vi "Find All New VIs.vi"(8 "error in":errorcluster, 10 "VIs  to exclude":variant) -> (0 "error out":errorcluster, 3 "VI refs":refnum<vi>[](array[refnum]))   [LabVIEW 2012, in "NI_SE_Config Front Panel Layout.lvlib"]
doc: "Find all VIs in memory that can be added to the layout configuration."
uses:
  NI_SE_Config Front Panel Layout.lvlib
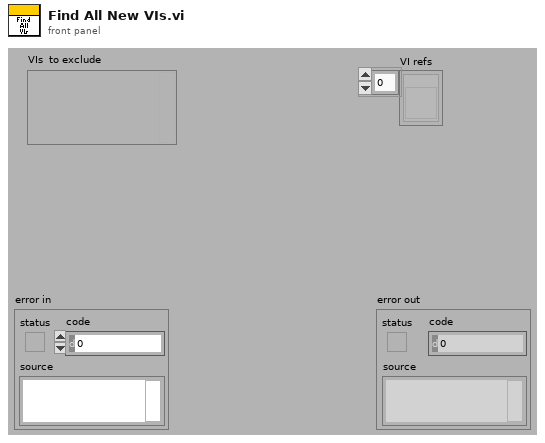
[diagram p1: front panel]
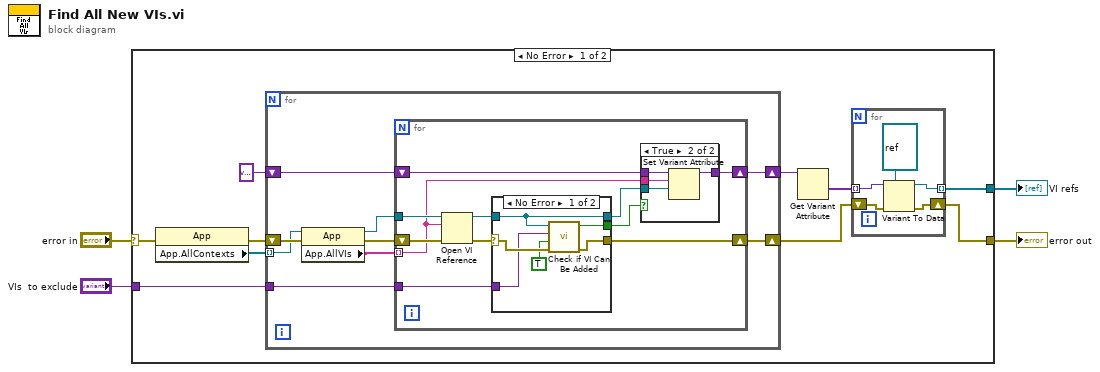
[diagram p0: block diagram]
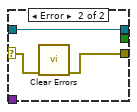
[diagram p3: hidden frame]
diagram:
  n1 = case shown="No Error" "error in" {
    selector: "error in" -> [w13 w54]
    tunnel: [w5 w54] -> w3
    tunnel: "VIs  to exclude" -> [w14 _]
    tunnel: [w7 _] -> w1
    frame No Error {
      n2 = property class="App"(error in=w13) -> (error out=w12:errorcluster, "App.AllContexts"=w11:refnum<vi>[])  [unwired: 1 in, 1 out]
      n3 = for {
        tunnel: w14 -> [w26]
        tunnel: w11 -> [w23] mode=indexing
        shift-right: [w25] -> w6
        shift-left: w12 -> [w24]
        shift-right: [w20] -> w9
        shift-left: variant ("variant") -> [w21]
        n4 = property class="App"(reference=w23, error in=w24) -> (reference out=w22:refnum<vi>, error out=w28:errorcluster, "App.AllVIs"=w27:string[])
        n5 = for {
          tunnel: w27 -> [w29] mode=indexing
          shift-right: [w38] -> w25
          shift-left: w28 -> [w39]
          tunnel: w26 -> [w35]
          tunnel: w22 -> [w32]
          shift-right: [w30] -> w20
          shift-left: w21 -> [w31]
          n6 = Open VI Reference(application reference (local)=w32, vi path=w29, error in (no error)=w39) -> (vi reference=w34:refnum<vi>, error out=w33:errorcluster)  [unwired: 3 in]
          n7 = case shown="No Error" w33 {
            selector: w33 -> [w50 w52]
            tunnel: w34 -> [w47 w53]
            tunnel: [w46 _] -> w36
            tunnel: [w49 w51] -> w38
            tunnel: [w47 w53] -> w37
            tunnel: w35 -> [w48 _]
            frame No Error {
              n8 = call "Check if VI Can Be Added.vi"("error in"=w50, "only accept open windows? (F)"=TRUE ("only accept open VIs? (F)"), "VIs to exclude"=w48, "VI refnum"=w47) -> ("error out"=w49:errorcluster, "allowed?"=w46:bool)  [unwired: 6 in]
            }
            frame Error {
              n9 = call <vilib>:"Clear Errors.vi"("error in (no error)"=w52) -> ("error out"=w51:errorcluster)  [unwired: 6 in]
            }
          }
          n10 = case shown="True" w36 {
            tunnel: w37 -> [_ w41]
            tunnel: w31 -> [w40 w44]
            tunnel: [w40 w43] -> w30
            tunnel: w29 -> [_ w42]
            frame False {
            }
            frame True {
              n11 = Set Variant Attribute(Variant=w44, name=w42, value=w41) -> (Variant out=w43:variant)  [unwired: 1 in, 2 out]
            }
          }
        }
      }
      n12 = Get Variant Attribute(Variant=w9) -> (values=w8:variant[])  [unwired: 3 in, 3 out]
      n13 = for {
        tunnel: w8 -> [w19] mode=indexing
        tunnel: [w17] -> w7 mode=indexing
        shift-right: [w16] -> w5
        shift-left: w6 -> [w15]
        n14 = Variant To Data(error in=w15, type=refnum<vi> refnum ("vi reference"), Variant=w19) -> (data=w17:refnum<vi>, error out=w16:errorcluster)
      }
    }
    frame Error {
    }
  }
  "error out" <- w3
  "VI refs" <- w1
